vi "Dir Folder With Attributes.vi"(7 "wildcard serach key (*)":string="*", 8 "error in (no error)":errorcluster, 9 "recoursive subfolders (/S)? (false)":bool, 10 "\"DIR /A:?\" attribute(s) (default: -H)":string="-H", 11 "folder":path) -> (0 "error out":errorcluster, 2 "file/folder paths":path[](array[path]), 3 "file/folder names":string[](array[string]))   [LabVIEW 2013]
doc: "Use Windows DIR command to list given folder content with filtering by attributes using [/A[:]] option of DIR. E.g. \"-H\" will list non hidden items only."
panel:
  out "standard output":string
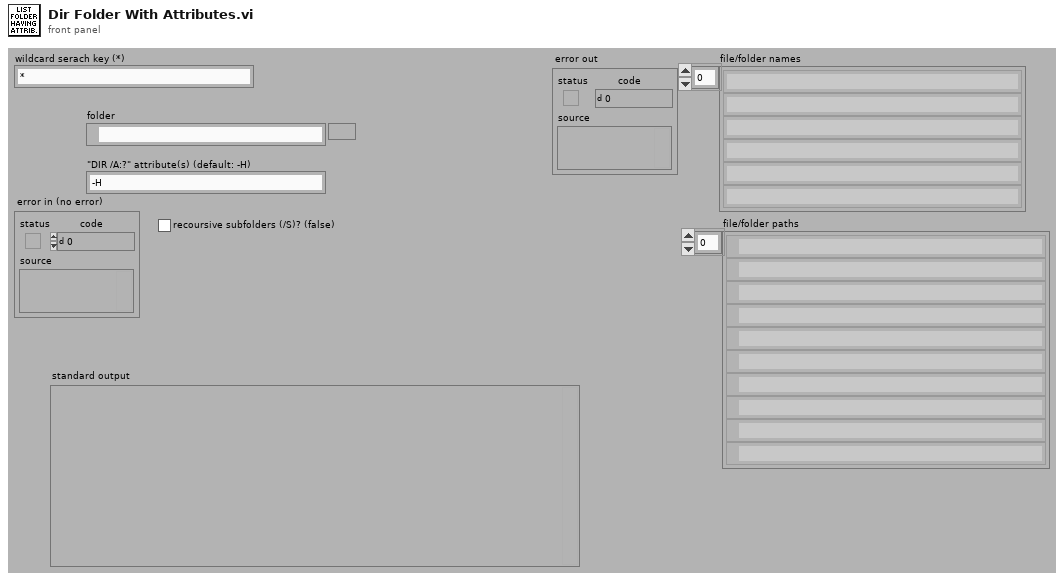
[diagram p1: front panel]
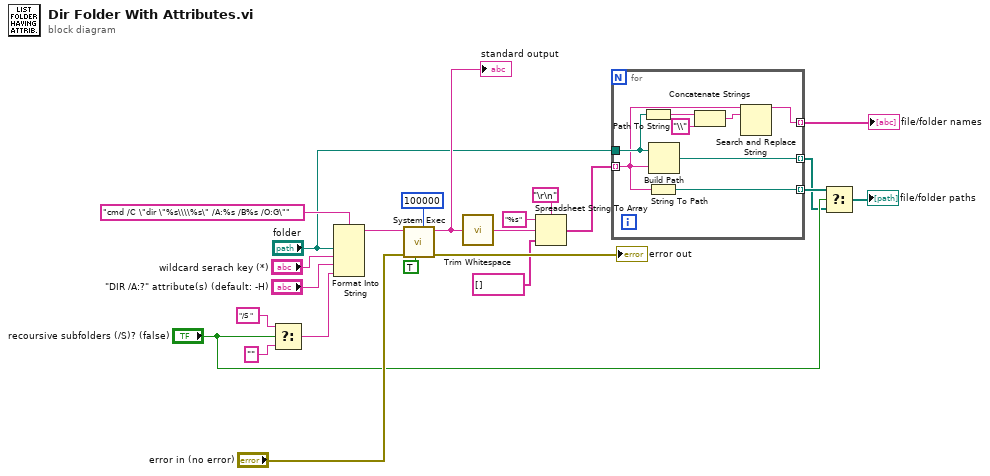
[diagram p0: block diagram]
diagram:
  n1 = Select(t="/S " ("format string"), s="recoursive subfolders (/S)? (false)", f="") -> (s? t:f=w7:string)
  n2 = Format Into String(format string="cmd /C \"dir \"%s\\\\%s\" /A:%s /B%s /O:G\"", "folder", "wildcard serach key (*)", "\"DIR /A:?\" attribute(s) (default: -H)", w7) -> (resulting string=w22:string)  [unwired: 2 in, 1 out]
  n3 = call <vilib>:"System Exec.vi"("expected output size  (4096)"=u32 100000, "run minimized? (F)"=TRUE, "error in (no error)"="error in (no error)", "command line"=w22) -> ("error out"=→"error out":errorcluster, "standard output"=w16:string)  [unwired: 4 in, 2 out]
  "standard output" <- w16
  n4 = call <vilib>:"Trim Whitespace.vi"("string"=w16) -> ("trimmed string"=w10:string)  [unwired: 1 in]
  n5 = Spreadsheet String To Array(delimiter (Tab)="\r\n", format string="%s", spreadsheet string=w10, array type (2D Dbl)=string[] []) -> (array=w12:string[])
  n6 = for {
    tunnel: w12 -> [w28] mode=indexing
    tunnel: "folder" -> [w29]
    tunnel: [w31] -> w3 mode=indexing
    tunnel: [w30] -> w4 mode=indexing
    tunnel: [w27] -> w1 mode=indexing
    n7 = Path To String(path=w29) -> (string=w26:string)
    n8 = String To Path(string=w28) -> (path=w30:path)
    n9 = Build Path(base path=w29, name or relative path=w28) -> (appended path=w31:path)
    n10 = Concatenate Strings(w26, "\\" ("string")) -> (w25:string)
    n11 = Search and Replace String(input string=w28, search string=w25) -> (result string=w27:string)  [unwired: 6 in, 3 out]
  }
  "file/folder names" <- w1
  n12 = Select(t=w4, s="recoursive subfolders (/S)? (false)", f=w3) -> (s? t:f=→"file/folder paths":path[])
